vi "pong for y (SubVI).vi"(7 "Numeric in":i32, 8 "y":i32, 11 "y szybkosc":i32) -> (0 "Numeric out":i32, 3 "y szybkosc wyjsciowa":i32)   [LabVIEW 2018]
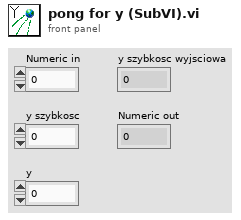
[diagram p1: front panel]
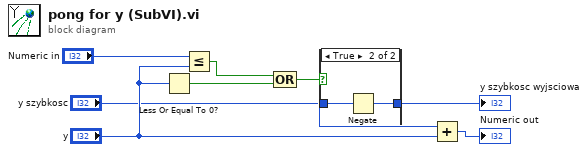
[diagram p0: block diagram]
diagram:
  n1 = Less Or Equal To 0?(x="y") -> (x <= 0?=w1:bool)
  n2 = Less Or Equal?(x="Numeric in", y="y") -> (x <= y?=w2:bool)
  n3 = Compound Arithmetic op=OR(w2, w1) -> (w3:bool)
  n4 = case shown="True" w3 {
    tunnel: "y szybkosc" -> [w9 w11]
    tunnel: [w9 w10] -> w6
    frame False {
    }
    frame True {
      n5 = Negate(x=w11) -> (-x=w10:i32)
    }
  }
  "y szybkosc wyjsciowa" <- w6
  n6 = Add(x=w6, y="y") -> (x+y=→"Numeric out":i32)
